vi "Create.vi"(5 "VolatusAPI":refnum<class "VolatusAPI.lvclass">, 7 "Variables":refnum<class "Variables.lvclass">, 11 "Source Name":string) -> (2 "error out":errorcluster, 3 "Condition Value out":refnum<class "Condition Value.lvclass">)   [LabVIEW 2020, in "VolatusSeq.lvlib" / "Condition Value.lvclass"]
uses:
  Condition Value.lvclass
  Variables/Variables.lvclass
  Volatus/VolatusAPI/VolatusAPI.lvclass
  Variables/Variables.lvclass/Variables.ctl
  Value Source.ctl
  Condition Value.lvclass/Condition Value.ctl
  Volatus/VolatusAPI/VolatusAPI.lvclass/VolatusAPI.ctl
  lv-vecto/Vecto/ChannelService/Lookup Double Channel.vi
  VolatusSeq.lvlib
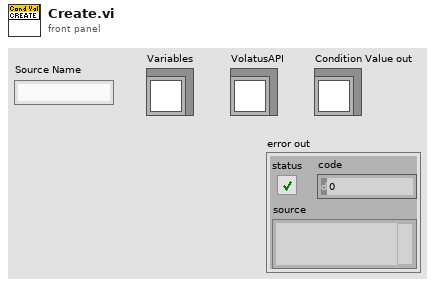
[diagram p1: front panel]
types:
  T1 = typedef "VolatusSeq.lvlib/Value Source.ctl" = enum16{"Channel", "Variable", "Expression"}
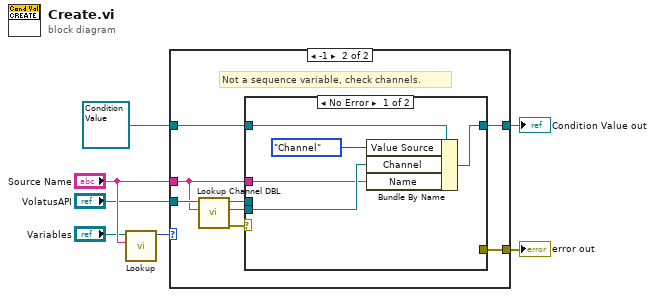
[diagram p0: block diagram]
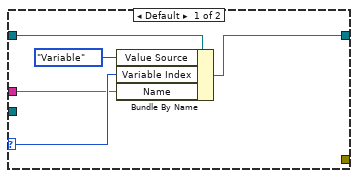
[diagram p2: hidden frame]
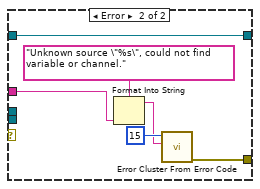
[diagram p3: hidden frame]
diagram:
  n1 = call "Lookup.vi"("Name"="Source Name", "Variables in"="Variables") -> ("Index"=w1:i32)  [unwired: 8 in, 1 out]
  n2 = case shown="-1" w1 {
    selector: w1 -> [w9 _]
    tunnel: refnum<class "Condition Value.lvclass"> refnum ("Condition Value in") -> [w12 w16]
    tunnel: [w10 w14] -> w3
    tunnel: "VolatusAPI" -> [_ w20]
    tunnel: "Source Name" -> [w8 w13]
    tunnel: [_ w15] -> w2
    frame Default {
      n3 = Bundle By Name(cluster=w12, "Value Source"=Value_Source."Variable", "Variable Index"=w9, "Name"=w8) -> (w10:refnum<class "Condition Value.lvclass">)
    }
    frame -1 {
      # "Not a sequence variable, check channels."
      n4 = call "Lookup Channel DBL.vi"("Name"=w13, "VolatusAPI in"=w20) -> ("error out"=w17:errorcluster, "Channel DBL"=w19:refnum<class "Channel DBL.lvclass">, "VolatusAPI out"=w18:refnum<class "VolatusAPI.lvclass">)  [unwired: 7 in]
      n5 = case shown="No Error" w17 {
        tunnel: w19 -> [w22 _]
        tunnel: w18 -> [_ _]
        tunnel: w16 -> [w25 w26]
        tunnel: [_ w29] -> w15
        tunnel: [w24 w26] -> w14
        tunnel: w13 -> [w21 w27]
        frame No Error {
          n6 = Bundle By Name(cluster=w25, "Value Source"=Value_Source."Channel", "Channel"=w22, "Name"=w21) -> (w24:refnum<class "Condition Value.lvclass">)
        }
        frame Error {
          n7 = Format Into String(format string="Unknown source \"%s\", could not find variable or channel.", w27) -> (resulting string=w30:string)  [unwired: 2 in, 1 out]
          n8 = call <vilib>:"Error Cluster From Error Code.vi"("error message (\"\")"=w30, "error code (0)"=15) -> ("error out"=w29:errorcluster)  [unwired: 7 in]
        }
      }
    }
  }
  "Condition Value out" <- w3
  "error out" <- w2
